vi "GPS Shutdown.vi"(11 "GPS COM port":refnum<visa-resource-name>) -> ()   [LabVIEW 2014]
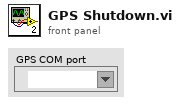
[diagram p1: front panel]
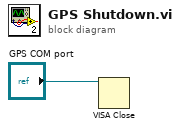
[diagram p0: block diagram]
diagram:
  n1 = VISA Close(VISA resource name="GPS COM port") -> ()  [unwired: 1 in, 1 out]
